vi "Set_Parameter_Instrument (Json).vi"(8 "error in (no error)":errorcluster caption="entrée d'erreur (pas d'erreur)", 10 "Parameter (Json)":string, 11 "Print_Label en entrée":refnum<class "Print_Label.lvclass">) -> (0 "error out":errorcluster caption="sortie d'erreur", 3 "Print_Label en sortie":refnum<class "Print_Label.lvclass">)   [LabVIEW 2020, in "Library Test.lvlib" / "Print_Label.lvclass"]
uses:
  Print_Label.lvclass
  C:/Users/ngarcin/OneDrive - Altyor/Standard TB/Class/Test/Test (Default)/Test (Default).lvclass
  Commun VI/TypeDef/Commande Printer/Commande Parameter Printer.ctl
  Printer/Printer (Default)/Class Printer (Default).lvclass
  JSON API/JSON Value/Set from JSON string.vi
  JSON API/Variant JSON/Variant to JSON.vi
  JSON API/JSON Value/Get Item by name array.vi
  Test_Wtih_Instr/Test_With_Inst.lvclass
  Instrument/Instrument (Default)/Class Instrument (Default).lvclass
  JSON API/JSON Value/JSON Value.lvclass
  Print_Label.lvclass/Print_Label.ctl
  JSON API/Variant JSON/Variant JSON.lvlib
  JSON API/Get Polymorphic/JSON GetSet.lvlib
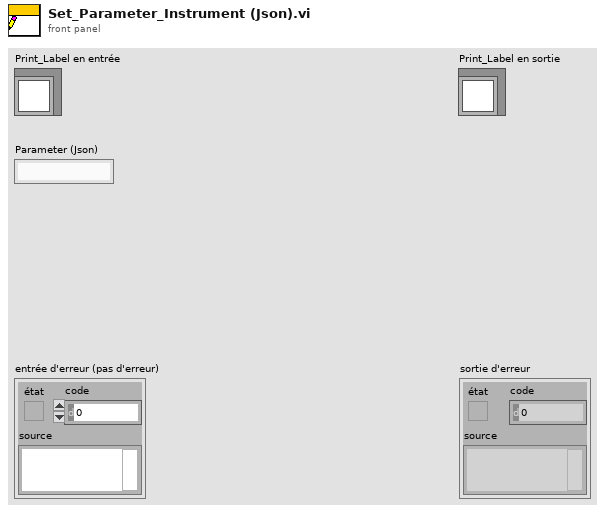
[diagram p1: front panel]
types:
  T1 = typedef "Commande Parameter Printer.ctl" = cluster{"Device_Printer":string, "File To print":path, "Path Picture":path, "Library Printer":refnum<class "Class Printer (Default).lvclass">}
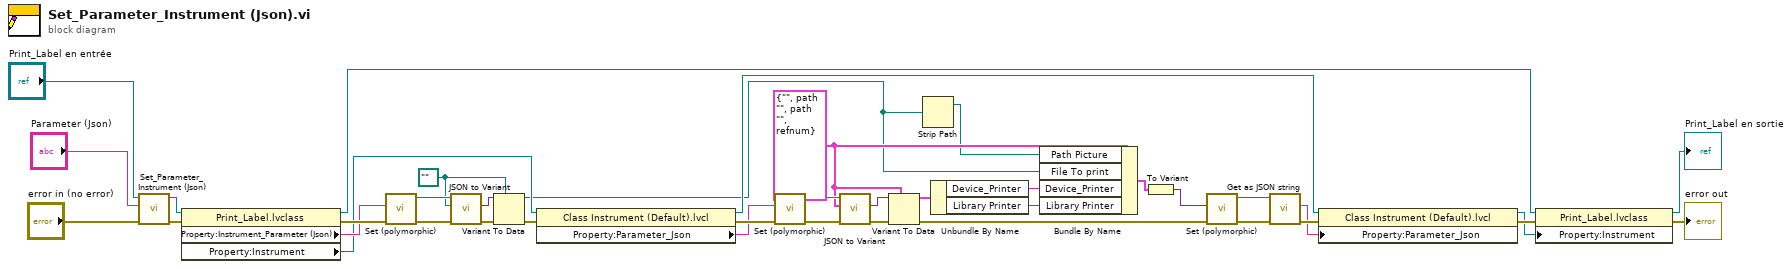
[diagram p0: block diagram]
diagram:
  w14 = path "" ("Path_Picture")
  w17 = T1 {"Device_Printer"="", "File To print"=path "", "Path Picture"=path "", "Library Printer"=refnum} ("Parameter")
  n1 = call-parent "Set_Parameter_Instrument (Json).vi"("error in (no error)"="error in (no error)", "Parameter (Json)"="Parameter (Json)", "Test (Default) en entrée"="Print_Label en entrée") -> ("error out"=w6:errorcluster, "Test (Default) en sortie"=w3:refnum<class "Print_Label.lvclass">)  [unwired: 7 in]
  n2 = property class="Print_Label.lvclass"(reference=w3, error in=w6) -> (reference out=w7:refnum<class "Print_Label.lvclass">, error out=w32:errorcluster, "Property:Instrument_Parameter (Json)"=w31:string, "Property:Instrument"=w29:refnum<class "Class Instrument (Default).lvclass">)
  n3 = call-poly "Set (polymorphic).vi"("error in (no error)"=w32, "JSON stream"=w31) -> ("error out"=w34:errorcluster, "JSON Value out"=w36:refnum<class "JSON Value.lvclass">)  [unwired: 7 in, 1 out]
  n4 = call "JSON to Variant.vi"("error in (no error)"=w34, "Variant (Data Type)"=w14, "JSON Value"=w36) -> ("error out"=w35:errorcluster, "Variant out"=w33:variant)  [unwired: 7 in]
  n5 = Variant To Data(error in=w35, type=w14, Variant=w33) -> (data=w2:path, error out=w30:errorcluster)
  n6 = property class="Class Instrument (Default).lvcl"(reference=w29, error in=w30) -> (reference out=w9:refnum<class "Class Instrument (Default).lvclass">, error out=w24:errorcluster, "Property:Parameter_Json"=w23:string)
  n7 = call-poly "Set (polymorphic).vi"("error in (no error)"=w24, "JSON stream"=w23) -> ("error out"=w27:errorcluster, "JSON Value out"=w25:refnum<class "JSON Value.lvclass">)  [unwired: 7 in, 1 out]
  n8 = call "JSON to Variant.vi"("error in (no error)"=w27, "Variant (Data Type)"=w17, "JSON Value"=w25) -> ("error out"=w26:errorcluster, "Variant out"=w28:variant)  [unwired: 7 in]
  n9 = Variant To Data(error in=w26, type=w17, Variant=w28) -> (data=w22:T1, error out=w18:errorcluster)
  n10 = Strip Path(path=w2) -> (stripped path=w1:path)  [unwired: 1 out]
  n11 = Unbundle By Name(w22) -> ("Device_Printer"=w16:string, "Library Printer"=w15:refnum<class "Class Printer (Default).lvclass">)
  n12 = Bundle By Name(cluster=w17, "Path Picture"=w1, "File To print"=w2, "Device_Printer"=w16, "Library Printer"=w15) -> (w13:T1)
  n13 = To Variant(anything=w13) -> (Variant=w21:variant)
  n14 = call-poly "Set (polymorphic).vi"("error in (no error)"=w18, "Variant"=w21) -> ("error out"=w19:errorcluster, "JSON Value out"=w20:refnum<class "JSON Value.lvclass">)  [unwired: 8 in]
  n15 = call "Get as JSON string.vi"("error in (no error)"=w19, "JSON Value in"=w20) -> ("error out"=w10:errorcluster, "<JSON>"=w8:string)  [unwired: 8 in]
  n16 = property class="Class Instrument (Default).lvcl"(reference=w9, error in=w10, "Property:Parameter_Json"=w8) -> (reference out=w11:refnum<class "Class Instrument (Default).lvclass">, error out=w12:errorcluster)
  n17 = property class="Print_Label.lvclass"(reference=w7, error in=w12, "Property:Instrument"=w11) -> (reference out=→"Print_Label en sortie":refnum<class "Print_Label.lvclass">, error out=→"error out":errorcluster)
